vi "JOG 테스트.vi"() -> ()   [LabVIEW 2014]
uses:
  <vilib>/DAQmx/create/channels.llb/DAQmx Create Channel (CO-Pulse Generation-Frequency).vi
  <vilib>/DAQmx/configure/timing.llb/DAQmx Timing (Implicit).vi
panel:
  in  "frequency":dbl=3600.0 caption="주파수" format="%.6f"
  in  "정지 버튼":bool
  in  "다음 버튼":bool
  in  "이전 버튼":bool
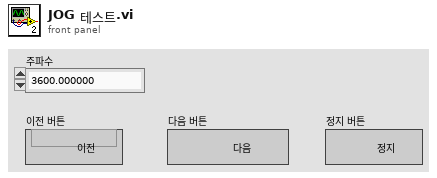
[diagram p1: front panel]
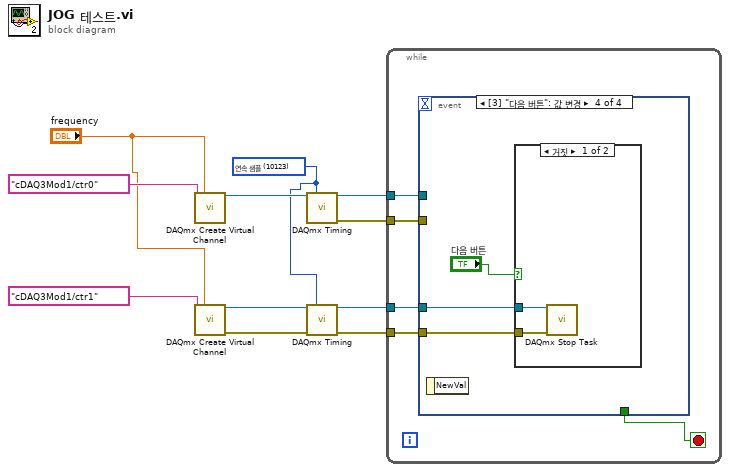
[diagram p0: block diagram]
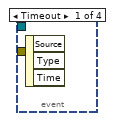
[diagram p2: hidden frame]
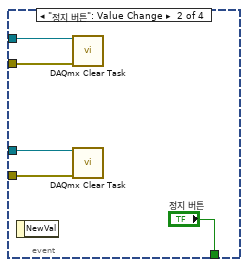
[diagram p3: hidden frame]
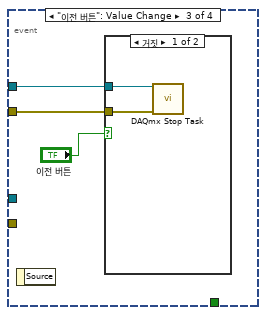
[diagram p4: hidden frame]
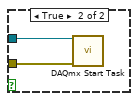
[diagram p5: hidden frame]
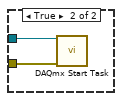
[diagram p6: hidden frame]
diagram:
  w7 = 10123 items=["유한 샘플"=10178, "연속 샘플"=10123, "하드웨어 타이밍에 의한 단일 포인트"=12522] ("sample mode")
  n1 = call-poly <vilib>:"DAQmx Create Virtual Channel.vi"("frequency"="frequency", "counter"=tag "cDAQ3Mod1/ctr0") -> ("task out"=w8:refnum<k21>)  [unwired: 12 in, 1 out]
  n2 = call-poly <vilib>:"DAQmx Create Virtual Channel.vi"("frequency"="frequency", "counter"=tag "cDAQ3Mod1/ctr1") -> ("task out"=w6:refnum<k21>, "error out"=w5:errorcluster)  [unwired: 12 in]
  n3 = call-poly <vilib>:"DAQmx Timing.vi"("task/channels in"=w8, "sample mode"=w7) -> ("task out"=w2:refnum<k21>, "error out"=w1:errorcluster)  [unwired: 12 in]
  n4 = call-poly <vilib>:"DAQmx Timing.vi"("task/channels in"=w6, "sample mode"=w7, "error in"=w5) -> ("task out"=w4:refnum<k21>, "error out"=w3:errorcluster)  [unwired: 11 in]
  n5 = while {
    tunnel: w4 -> [w15]
    tunnel: w3 -> [w14]
    tunnel: w2 -> [w13]
    tunnel: w1 -> [w12]
    stop <- w16 stop-if-true
    n6 = event shown="[3] \"다음 버튼\": 값 변경" {
      selector: _ -> [_ _ _ _]
      dyn-events: _ -> [_ _ _ _]
      timeout: _ -> [_ _ _ _]
      tunnel: [_ "정지 버튼" _ _] -> w16
      tunnel: w15 -> [_ w20 _ w30]
      tunnel: w14 -> [_ w19 _ w29]
      tunnel: w13 -> [_ w18 w23 _]
      tunnel: w12 -> [_ w17 w22 _]
      event Timeout {
        n7 = event-data() -> ()  [unwired: 1 in, 3 out]
      }
      event "정지 버튼": Value Change {
        n8 = event-data() -> ()  [unwired: 1 in, 1 out]
        n9 = call <vilib>:"DAQmx Clear Task.vi"("task in"=w18, "error in"=w17) -> ()  [unwired: 13 in, 1 out]
        n10 = call <vilib>:"DAQmx Clear Task.vi"("task in"=w20, "error in"=w19) -> ()  [unwired: 13 in, 1 out]
      }
      event "이전 버튼": Value Change {
        n11 = event-data() -> ()  [unwired: 1 in, 1 out]
        n12 = case shown="거짓" "이전 버튼" {
          tunnel: w23 -> [w26 w28]
          tunnel: w22 -> [w25 w27]
          frame False {
            n13 = call <vilib>:"DAQmx Stop Task.vi"("task/channels in"=w26, "error in"=w25) -> ()  [unwired: 12 in, 2 out]
          }
          frame True {
            n14 = call <vilib>:"DAQmx Start Task.vi"("task/channels in"=w28, "error in"=w27) -> ()  [unwired: 12 in, 2 out]
          }
        }
      }
      event "다음 버튼": Value Change {
        n15 = event-data() -> ()  [unwired: 1 in, 1 out]
        n16 = case shown="거짓" "다음 버튼" {
          tunnel: w30 -> [w33 w35]
          tunnel: w29 -> [w32 w34]
          frame False {
            n17 = call <vilib>:"DAQmx Stop Task.vi"("task/channels in"=w33, "error in"=w32) -> ()  [unwired: 12 in, 2 out]
          }
          frame True {
            n18 = call <vilib>:"DAQmx Start Task.vi"("task/channels in"=w35, "error in"=w34) -> ()  [unwired: 12 in, 2 out]
          }
        }
      }
    }
  }
